vi "Start Action Core.vi"(8 "error in (no error)":errorcluster, 11 "NI DAQmx AI Voltage in":refnum<class "NI DAQmx AI Voltage.lvclass">) -> (0 "error out":errorcluster, 3 "NI DAQmx AI Voltage out":refnum<class "NI DAQmx AI Voltage.lvclass">)   [LabVIEW 2020, in "NI DAQmx AI Voltage.lvlib" / "NI DAQmx AI Voltage.lvclass"]
uses:
  NI DAQmx AI Voltage.lvclass
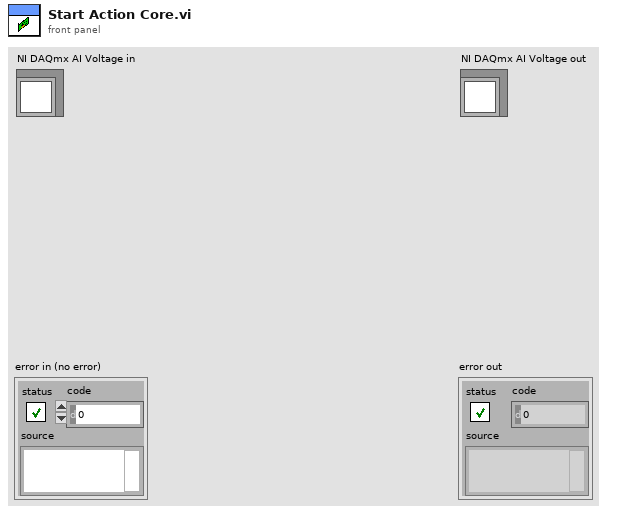
[diagram p1: front panel]
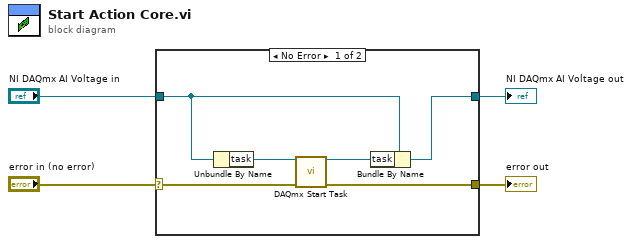
[diagram p0: block diagram]
diagram:
  n1 = case shown="No Error" "error in (no error)" {
    selector: "error in (no error)" -> [w10 w12]
    tunnel: "NI DAQmx AI Voltage in" -> [w8 w11]
    tunnel: [w7 w12] -> w2
    tunnel: [w5 w11] -> w1
    frame No Error {
      n2 = Unbundle By Name(w8) -> ("task"=w9:refnum<k21>)
      n3 = call <vilib>:"DAQmx Start Task.vi"("task/channels in"=w9, "error in"=w10) -> ("task out"=w6:refnum<k21>, "error out"=w7:errorcluster)  [unwired: 12 in]
      n4 = Bundle By Name(cluster=w8, "task"=w6) -> (w5:refnum<class "NI DAQmx AI Voltage.lvclass">)
    }
    frame Error {
    }
  }
  "error out" <- w2
  "NI DAQmx AI Voltage out" <- w1
